vi "XSP3_PutI32.vi"(6 "I32":i32, 8 "ErrorIn":errorcluster, 9 "Time":dbl=1.0 caption="TimeOut/s", 10 "Wait":u32=10 caption="Wait/ms", 11 "PVIn":string caption="PVNameIn") -> (0 "ErrorOut":errorcluster, 2 "Status":bool, 3 "PVOut":string caption="PVNameOut", 4 "PVError":errorcluster)   [LabVIEW 2010]
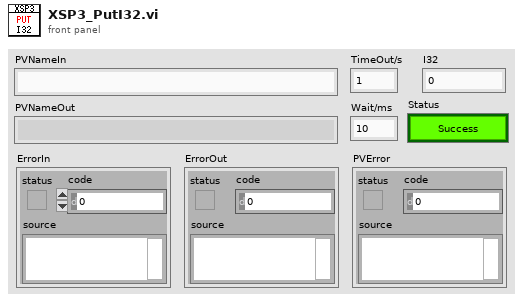
[diagram p1: front panel]
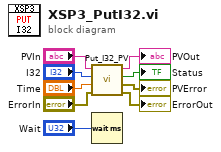
[diagram p0: block diagram]
diagram:
  n1 = call "Put_I32_PV.vi"("Error in (no error)"="ErrorIn", "Timeout (3)"="Time", "Value"="I32", "PV Name"="PVIn") -> ("Error out"=→"ErrorOut":errorcluster, "PV error"=→"PVError":errorcluster, "Status"=→"Status":bool, "PV Name (dup)"=→"PVOut":string)  [unwired: 4 in]
  n2 = Wait (ms)(milliseconds to wait="Wait") -> ()  [unwired: 1 out]
